vi "Task ID.vi"(8 "error in (no error)":errorcluster, 11 "SimTask in":refnum<class "SimTask.lvclass">) -> (0 "error out":errorcluster, 2 "Task ID":string, 3 "SimTask out":refnum<class "SimTask.lvclass">)   [LabVIEW 2020, in "VolatusDemo.lvlib" / "SimTask.lvclass"]
uses:
  SimTask.lvclass
  SimTask.lvclass/SimTask.ctl
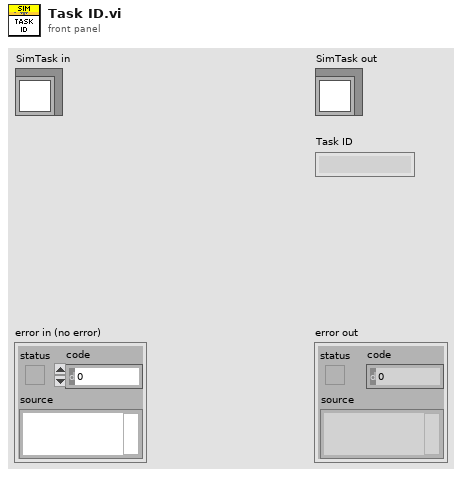
[diagram p1: front panel]
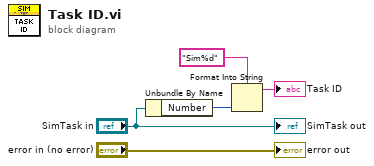
[diagram p0: block diagram]
diagram:
  n1 = Unbundle By Name("SimTask in") -> ("Number"=w3:i32)
  n2 = Format Into String(format string="Sim%d", w3) -> (resulting string=→"Task ID":string)  [unwired: 2 in, 1 out]
  "error out" <- "error in (no error)"
  "SimTask out" <- "SimTask in"
